vi "parse_pose_roslv.vi"(4 "error in":errorcluster, 7 "msg in":string) -> (0 "error out":errorcluster, 2 "Pose":T1, 3 "msg out":string)   [LabVIEW 2014]
doc: "Parses a message into a pose"
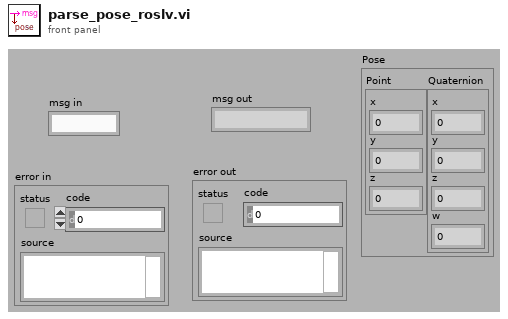
[diagram p1: front panel]
types:
  T1 = cluster{"Point":cluster{"x":dbl, "y":dbl, "z":dbl}, "Quaternion":cluster{"x":dbl, "y":dbl, "z":dbl, "w":dbl}}
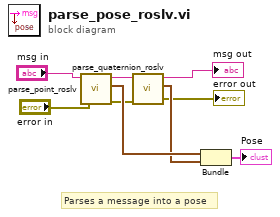
[diagram p0: block diagram]
diagram:
  # "Parses a message into a pose"
  n1 = call "parse_point_roslv.vi"("error in"="error in", "msg in"="msg in") -> ("error out"=w3:errorcluster, "Point"=w6:cluster{"x":dbl, "y":dbl, "z":dbl}, "msg out"=w9:string)  [unwired: 3 in]
  n2 = call "parse_quaternion_roslv.vi"("error in"=w3, "msg in"=w9) -> ("error out"=→"error out":errorcluster, "Quaternion"=w5:cluster{"x":dbl, "y":dbl, "z":dbl, "w":dbl}, "msg out"=→"msg out":string)  [unwired: 3 in]
  n3 = Bundle("Point"=w6, "Quaternion"=w5) -> (→"Pose":T1)  [unwired: 1 in]
